vi "Get Matrix from Transform.vi"(1 "Transform Attributes":string[](array[string])) -> (0 "Matrix":T1)   [LabVIEW 2013]
doc: "This VI parses an array of transform attributes into a transformation matrix. If the transform element is a matrix, it reads [a b c d e f] directly into an array. If the transform element is a translate, it puts the translate data into the correct matrix elements. More information about transform matrices can be found in the SVG 1.1 Specifications: http://www.w3.org/TR/SVG11/"
uses:
  <vilib>/Analysis/Matrix/Datatypes/RealMatrix.ctl
  <vilib>/Analysis/Matrix/Numeric/Conversions/Array To Matrix - RA2.vi
  <vilib>/Analysis/Matrix/NI_Matrix.lvlib
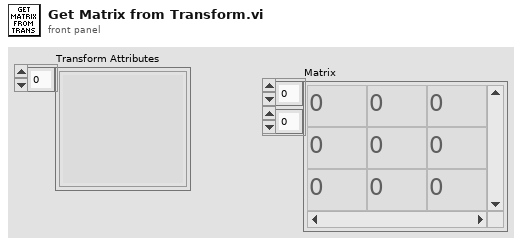
[diagram p1: front panel]
types:
  T1 = typedef "NI_Matrix.lvlib/RealMatrix.ctl" = dbl[][]
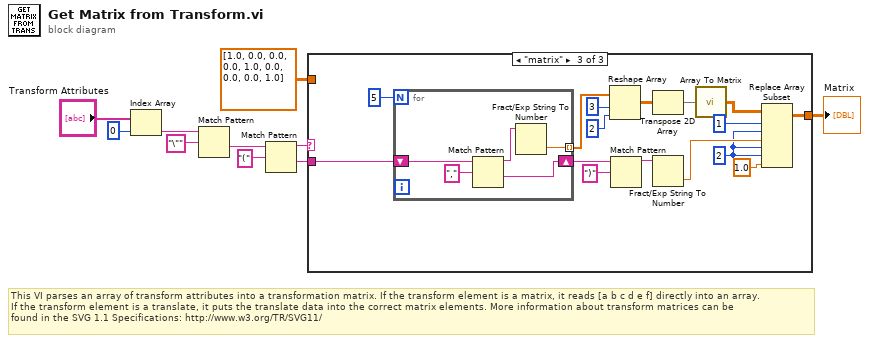
[diagram p0: block diagram]
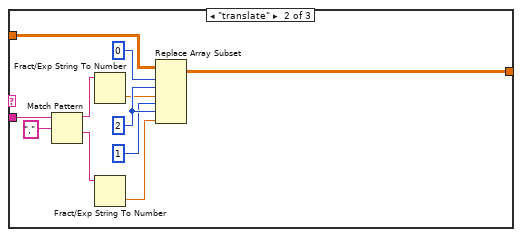
[diagram p3: hidden frame]
diagram:
  # "This VI parses an array of transform attributes into a transformation matrix. If the transform element is a matrix, it reads [a b c d e f] directly into an array. \nIf the transform element is a translate, it puts the translate data into the correct matrix elements. More information about transform matrices can be\nfound in the SVG 1.1 Specifications: http://www.w3.org/TR/SVG11/"
  n1 = Index Array(array="Transform Attributes", index=0) -> (element=w3:string)
  n2 = Match Pattern(string=w3, regular expression="\"") -> (after substring=w4:string)  [unwired: 1 in, 3 out]
  n3 = Match Pattern(string=w4, regular expression="(") -> (before substring=w1:string, after substring=w8:string)  [unwired: 1 in, 2 out]
  n4 = case shown="\"matrix\"" w1 {
    tunnel: w8 -> [_ w21 w38]
    tunnel: [w11 w12 w25] -> w10
    tunnel: T1 [[1.0, 0.0, 0.0], [0.0, 1.0, 0.0], [0.0, 0.0, 1.0]] ("matrix") -> [w11 w13 _]
    frame "", Default {
    }
    frame "translate" {
      w18 = 2 ("index (col)")
      n5 = Match Pattern(string=w21, regular expression=",") -> (before substring=w20:string, after substring=w19:string)  [unwired: 1 in, 2 out]
      n6 = Fract/Exp String To Number(string=w20) -> (number=w14:dbl)  [unwired: 3 in, 1 out]
      n7 = Fract/Exp String To Number(string=w19) -> (number=w15:dbl)  [unwired: 3 in, 1 out]
      n8 = Replace Array Subset(array=w13, new element #1=w14, index (row) #1=0 ("disabled index (row)"), index (col) #1=w18, new element #2=w15, index (row) #2=1 ("disabled index (row)"), index (col) #2=w18) -> (w12:T1)
    }
    frame "matrix" {
      w24 = 2 ("disabled index (col)")
      n9 = for {
        N: 5 -> [_]
        tunnel: [w40] -> w32 mode=indexing
        shift-right: [w39] -> w36
        shift-left: w38 -> [w42]
        n10 = Match Pattern(string=w42, regular expression=",") -> (before substring=w41:string, after substring=w39:string)  [unwired: 1 in, 2 out]
        n11 = Fract/Exp String To Number(string=w41) -> (number=w40:dbl)  [unwired: 3 in, 1 out]
      }
      n12 = Reshape Array(w32, 3 ("dimension size"), 2 ("dimension size")) -> (w27:dbl[][])
      n13 = Match Pattern(string=w36, regular expression=")") -> (before substring=w34:string)  [unwired: 1 in, 3 out]
      n14 = Transpose 2D Array(2D array=w27) -> (transposed array=w26:dbl[][])
      n15 = Fract/Exp String To Number(string=w34) -> (number=w28:dbl)  [unwired: 3 in, 1 out]
      n16 = call-poly <vilib>:"Array To Matrix.vi"("Real 2D Array"=w26) -> ("Real Matrix"=w30:T1)
      n17 = Replace Array Subset(array=w30, new element #1=w28, index (row) #1=1 ("disabled index (row)"), index (col) #1=w24, new element #2=1.0 ("new element/submatrix"), index (row) #2=w24, index (col) #2=w24) -> (w25:T1)
    }
  }
  "Matrix" <- w10
